vi "Actor Core.vi"(8 "error in":errorcluster, 11 "Controller in":refnum<class "Controller.lvclass">) -> (0 "error out":errorcluster, 3 "Actor out":refnum<class "Actor.lvclass">)   [LabVIEW 2016, in "Controller Actor.lvlib" / "Controller.lvclass"]
doc: "(<B>Filename</B>: Actor Framework.lvlib:Actor.lvclass:Actor Core.vi)\n\nReceives messages to the actor, reacts to them, and initiates any error handling that may shut the actor down.\n\nDescendant classes may override this VI to append parallel tasks for the actor to complete while it handles messages. Overrides use the Call Parent Method node."
uses:
  Controller.lvclass
  <vilib>/ActorFramework/Actor/Actor.lvclass
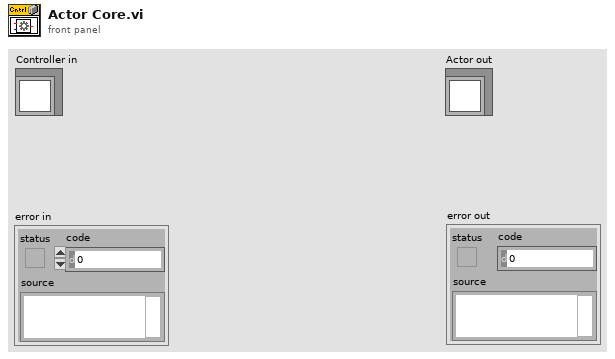
[diagram p1: front panel]
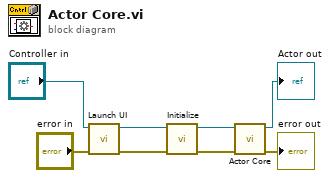
[diagram p0: block diagram]
diagram:
  n1 = call-dynamic "Launch UI.vi"("error in (no error)"="error in", "Controller In"="Controller in") -> ("error out"=w1:errorcluster, "Controller Out"=w3:refnum<class "Controller.lvclass">)  [unwired: 8 in]
  n2 = call-dynamic "Initialize.vi"("error in (no error)"=w1, "Controller Actor.lvlib:Controller.lvclass"=w3) -> ("error out"=w5:errorcluster, "Controller out"=w6:refnum<class "Controller.lvclass">)  [unwired: 8 in]
  n3 = call-parent "Actor Core.vi"("error in"=w5, "Actor in"=w6) -> ("error out"=→"error out":errorcluster, "Actor out"=→"Actor out":refnum<class "Actor.lvclass">)  [unwired: 8 in]
